vi "SetExternalInterfaces.vi"(8 "Error In":errorcluster, 10 "ExternalInterfaces":T1[](array[typedef]), 11 "reference in":refnum<class "VerticalButtonBar.lvclass">) -> (0 "Error Out":errorcluster, 3 "reference in":refnum<class "VerticalButtonBar.lvclass">)   [LabVIEW 2021, in "VerticalButtonBar.lvclass"]
uses:
  VerticalButtonBar.lvclass
  .Externals/Library_TAF_Support/ClusterArrayConversion/BundledArray.ctl
  0a6ec689-4898-488c-8e07-ed5616c8d135.vi
  0a6ec689-4898-488c-8e07-ed5616c8d135.vi/e733eca7-9823-4359-8665-3b184f9a7377.vi
  0a6ec689-4898-488c-8e07-ed5616c8d135.vi/185eb5ab-e8f7-4395-854b-f566a9b9020c.vi
  <vilib>/Utility/Data Type/Get Cluster Information.vi
  <vilib>/Utility/Data Type/Get Type Information.vi
  <userlib>/_OpenG.lib/lvdata/lvdata.llb/Array of VData to VCluster__ogtk.vi
  <vilib>/Utility/LVClass/Get LV Class Name.vi
  .Externals/Library_TAF_Support/ClusterArrayConversion/ClusterArrayConversion.lvlib
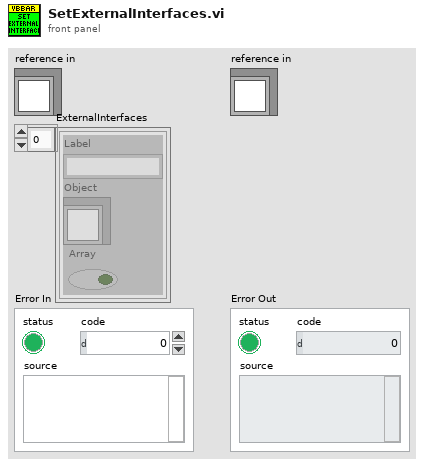
[diagram p1: front panel]
types:
  T1 = typedef "ClusterArrayConversion.lvlib/BundledArray.ctl" = cluster{"Label":string, "Object":refnum<class>, "Array":bool}
  T2 = typedef "VerticalButtonBar.lvclass/ObjectAttributes.ctl" = cluster{"Interfaces":cluster{"IDockGUI":refnum<class "IDockGUI.lvclass">, "Authorizer":refnum<class "IAuthorization.lvclass">}, "Locals":cluster{"ButtonBar":refnum<class "ButtonCollection.lvclass">, "BaseConfigurationPath":path, "Labels":cluster{"Label":string, "Value":string}[]}, "Persistent":cluster{"ButtonDefinitionFile":string}}
  T3 = cluster{"IDockGUI":refnum<class "IDockGUI.lvclass">, "Authorizer":refnum<class "IAuthorization.lvclass">}
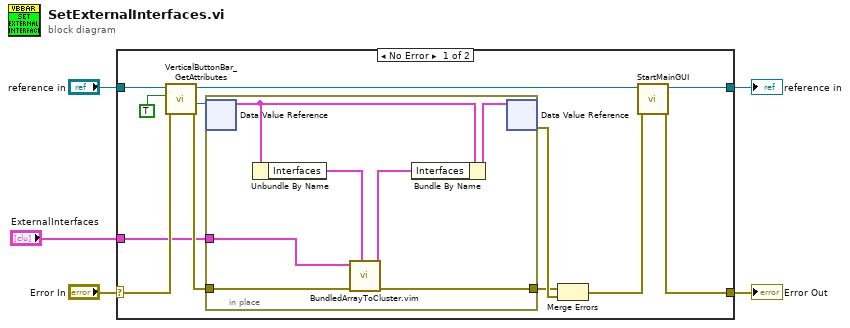
[diagram p0: block diagram]
diagram:
  n1 = case shown="No Error" "Error In" {
    selector: "Error In" -> [w15 w26]
    tunnel: [w6 w26] -> w4
    tunnel: [w8 w25] -> w2
    tunnel: "reference in" -> [w17 w25]
    tunnel: "ExternalInterfaces" -> [w9 _]
    frame No Error {
      n2 = call "VerticalButtonBar_GetAttributes.vi"("error in (no error)"=w15, "OnlyGetDvrReference(False)"=TRUE, "reference in"=w17) -> ("error out"=w10:errorcluster, "DataRef"=w12:refnum<data-value>, "reference out"=w16:refnum<class "VerticalButtonBar.lvclass">)  [unwired: 5 in, 1 out]
      n3 = in-place {
        in-place-border: [w23] -> w11
        in-place-border: w10 -> [w20]
        in-place-border: w9 -> [w21]
        n4 = in-place-dvr #1(w12) -> (w22:T2)  [unwired: 1 out]
        n5 = Unbundle By Name(w22) -> ("Interfaces"=w19:T3)
        n6 = call "BundledArrayToCluster.vim"("Type"=w19, "error in (no error)"=w20, "BundeledLabels"=w21) -> ("error out"=w23:errorcluster, "DataOut"=w18:T3)  [unwired: 7 in]
        n7 = Bundle By Name(cluster=w22, "Interfaces"=w18) -> (w24:T2)
        n8 = in-place-dvr #1(w24) -> (w13:errorcluster)  [unwired: 1 out]
      }
      n9 = Merge Errors(w11, w13) -> (w7:errorcluster)
      n10 = call "StartMainGUI.vi"("Error In"=w7, "reference in"=w16) -> ("Error Out"=w6:errorcluster, "reference out"=w8:refnum<class "VerticalButtonBar.lvclass">)  [unwired: 6 in, 2 out]
    }
    frame Error {
    }
  }
  "Error Out" <- w4
  "reference in" <- w2
